vi "WaitForTemp.vi"(8 "error out":errorcluster, 10 "Setpoint":i32=-20) -> (0 "error out 2":errorcluster)   [LabVIEW 2018, in "Andor Camera.lvlib"]
uses:
  Andor Camera.lvlib
panel:
  in  "STOP":bool
  out "Please wait for camera temperature to reach setpoint...":i32
  # "C"
  # "C"
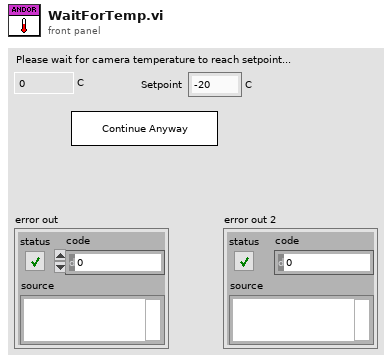
[diagram p1: front panel]
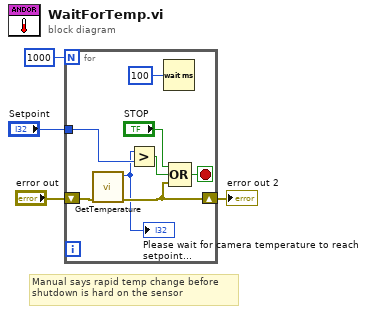
[diagram p0: block diagram]
diagram:
  # "Manual says rapid temp change before\nshutdown is hard on the sensor"
  n1 = for {
    N: 1000 -> [_]
    shift-right: [w7] -> w2
    shift-left: "error out" -> [w12]
    tunnel: "Setpoint" -> [w6]
    stop <- w10 stop-if-true
    n2 = call <userlib>:"GetTemperature.vi"("error in (no error)"=w12) -> ("error out"=w7:errorcluster, "temperature"=w5:i32)  [unwired: 3 in, 2 out]
    "Please wait for camera temperature to reach setpoint..." <- w5
    n3 = Greater?(x=w5, y=w6) -> (0:w8:bool)
    n4 = Wait (ms)(milliseconds to wait=u32 100) -> ()  [unwired: 1 out]
    n5 = Compound Arithmetic op=OR("STOP", w8, w7) -> (w10:bool)
  }
  "error out 2" <- w2
